vi "ElevatorButtonsTest.vi"() -> ()   [LabVIEW 2018]
panel:
  out "State":i32
  in  "State 3":bool
  in  "State 2":bool
  in  "State 1":bool
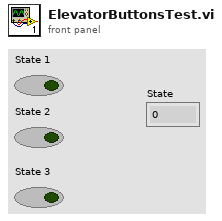
[diagram p1: front panel]
types:
  T1 = cluster{"State 1":bool, "State 2":bool, "State 3":bool}
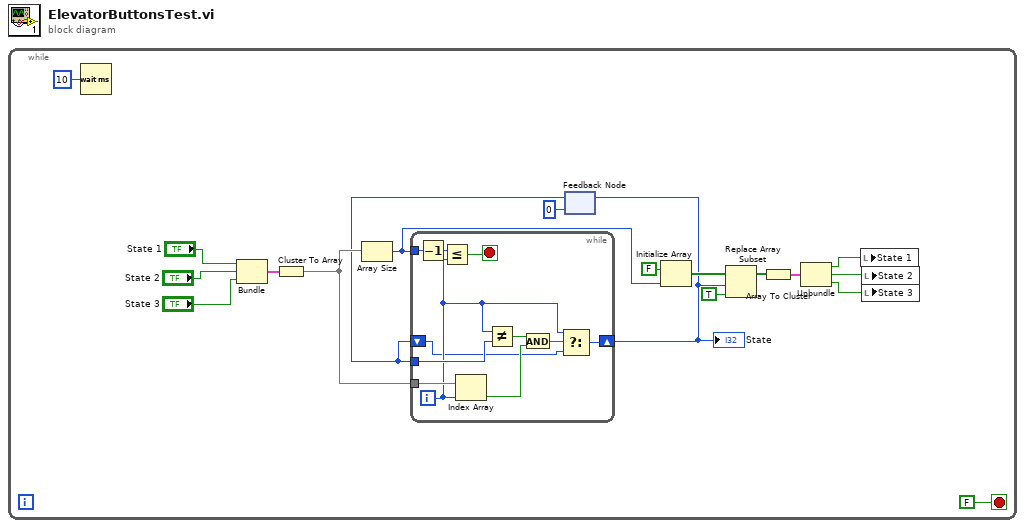
[diagram p0: block diagram]
diagram:
  n1 = while {
    stop <- FALSE stop-if-true
    n2 = Wait (ms)(milliseconds to wait=u32 10) -> ()  [unwired: 1 out]
    n3 = Bundle("State 1"="State 1", "State 2"="State 2", "State 3"="State 3") -> (w16:T1)  [unwired: 1 in]
    n4 = Cluster To Array(cluster=w16) -> (array=w15:bool[])
    n5 = Array Size(array=w15) -> (size(s)=w12:i32)
    n6 = feedback #1(0) -> (w13:i32)
    n7 = while {
      tunnel: w15 -> [w30]
      tunnel: w13 -> [w25]
      tunnel: w12 -> [w23]
      shift-right: [w26] -> w9
      shift-left: w13 -> [w20]
      i -> [w24]
      stop <- w22 stop-if-true
      n8 = Decrement(x=w23) -> (x-1=w21:i32)
      n9 = Less Or Equal?(x=w21, y=w24) -> (x <= y?=w22:bool)
      n10 = Index Array(array=w30, index=w24) -> (element=w28:bool)
      n11 = Not Equal?(x=w24, y=w25) -> (x != y?=w27:bool)
      n12 = And(x=w27, y=w28) -> (x .and. y?=w29:bool)
      n13 = Select(t=w24, s=w29, f=w20) -> (s? t:f=w26:i32)
    }
    "State" <- w9
    n14 = feedback-in #1(w9) -> ()
    n15 = Initialize Array(FALSE, w12) -> (w10:bool[])
    n16 = Replace Array Subset(array=w10, new element=TRUE ("new element/subarray"), index=w9) -> (w7:bool[])
    n17 = Array To Cluster(array=w7) -> (cluster=w6:cluster{"[0]":bool, "[1]":bool, "[2]":bool})
    n18 = Unbundle(w6) -> ("[0]"=w3:bool, "[1]"=w2:bool, "[2]"=w1:bool)
    n19 = local write "State 1"(w3) -> ()
    n20 = local write "State 2"(w2) -> ()
    n21 = local write "State 3"(w1) -> ()
  }
